vi "Script Property Global into VI.vi"(4 "GlobalControlName":string="Compiled.Settings", 6 "StringConstantToReplace":string="Compiled.Settings", 8 "error in (no error)":errorcluster, 10 "Path to Global":path, 11 "Path to VI":path) -> (0 "error out":errorcluster)   [LabVIEW 2015]
doc: "This VI replaces a string constant in the template, by name, with a string global by name and path."
uses:
  <vilib>/Utility/traverseref.llb/TRef TravTarget.ctl
  <vilib>/Utility/traverseref.llb/VI Scripting - Traverse.lvlib
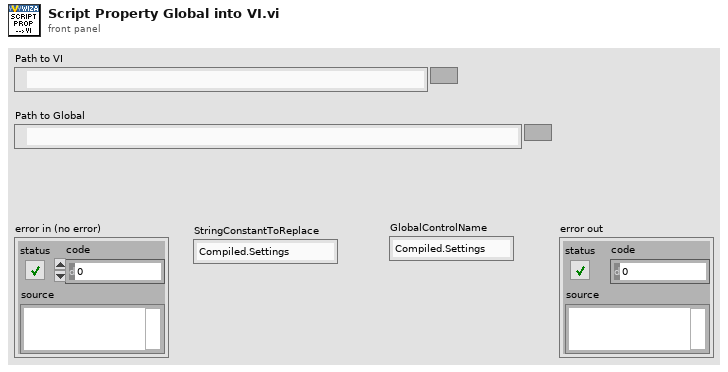
[diagram p1: front panel]
types:
  T1 = typedef "TRef TravTarget.ctl" = enum16{"FP", "BD", "Other"}
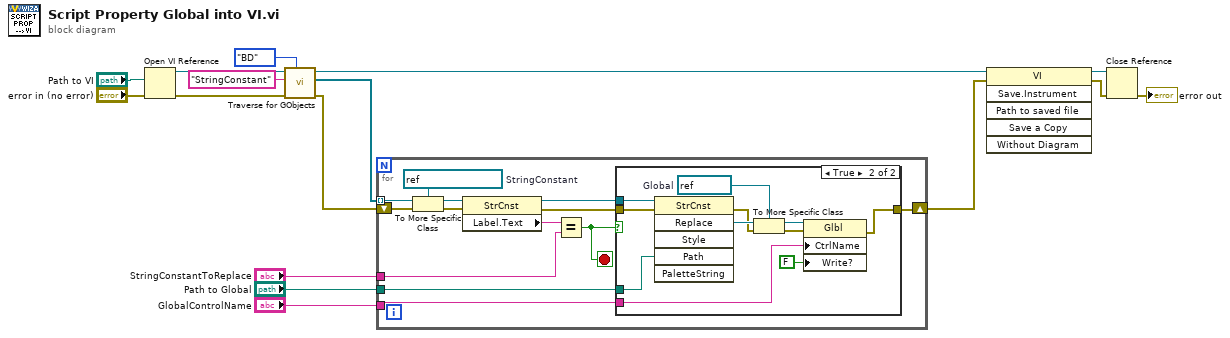
[diagram p0: block diagram]
diagram:
  n1 = Open VI Reference(vi path="Path to VI", error in (no error)="error in (no error)") -> (vi reference=w8:refnum<vi>, error out=w9:errorcluster)  [unwired: 4 in]
  n2 = call <vilib>:"Traverse for GObjects.vi"("Traverse Target"=TRef_TravTarget."BD", "error in (no error)"=w9, "Class Name"="StringConstant", "VI Refnum"=w8) -> ("error out"=w4:errorcluster, "References"=w3:refnum<vi>[], "dup VI Refnum"=w10:refnum<vi>)  [unwired: 4 in, 1 out]
  n3 = for {
    tunnel: w3 -> [w29] mode=indexing
    shift-right: [w20] -> w14
    shift-left: w4 -> [w27]
    tunnel: "StringConstantToReplace" -> [w18]
    tunnel: "Path to Global" -> [w21]
    tunnel: "GlobalControlName" -> [w17]
    stop <- w19 stop-if-true
    w28 = refnum<vi> refnum  # StringConstant
    n4 = To More Specific Class(target class=w28, reference=w29, error in=w27) -> (specific class reference=w26:refnum<vi>, error out=w25:errorcluster)
    n5 = property class="StrCnst"(reference=w26, error in=w25) -> (reference out=w23:refnum<vi>, error out=w22:errorcluster, "Label.Text"=w24:string)
    n6 = Equal?(x=w24, y=w18) -> (x = y?=w19:bool)
    n7 = case shown="True" w19 {
      tunnel: w23 -> [_ w41]
      tunnel: w22 -> [w30 w40]
      tunnel: w21 -> [_ w39]
      tunnel: [w30 w32] -> w20
      tunnel: w17 -> [_ w33]
      frame False {
      }
      frame True {
        w36 = refnum<vi> refnum  # Global
        n8 = invoke class="StrCnst" method="Replace"(reference=w41, error in=w40, "Path"=w39) -> (error out=w37:errorcluster, "Replace"=w38:refnum<vi>)  [unwired: 3 in, 4 out]
        n9 = To More Specific Class(target class=w36, reference=w38, error in=w37) -> (specific class reference=w35:refnum<vi>, error out=w34:errorcluster)
        n10 = property class="Glbl"(reference=w35, error in=w34, "CtrlName"=w33, "Write?"=FALSE) -> (error out=w32:errorcluster)  [unwired: 1 out]
      }
    }
  }
  n11 = invoke class="VI" method="Save.Instrument"(reference=w10, error in=w14) -> (reference out=w11:refnum<vi>, error out=w12:errorcluster)  [unwired: 4 in, 4 out]
  n12 = Close Reference(reference=w11, error in (no error)=w12) -> (error out=→"error out":errorcluster)
